vi "Begin.vi"(11 "Image Size":T1=enum."160x120") -> (0 "error out":errorcluster)   [LabVIEW 2012]
doc: "Called before other user functions, this VI is expected to open initial I/O refnums, load in file data, and do all program initialization. Notice that the <B>error out</B> terminal is simply used for data flow. Wiring it to other structures or subVIs ensures that this VI runs first."
uses:
  <vilib>/Rock Robotics/WPI/Camera/WPI_CameraImageSize.ctl
  <vilib>/Rock Robotics/SystemInterfaces/DIO/FPGA_DIOPWMChannel.ctl
  <vilib>/Rock Robotics/WPI/Joystick/WPI_JoystickDeviceEnum.ctl
  <vilib>/Rock Robotics/SystemInterfaces/DIO/FPGA_DIOChannel.ctl
  <vilib>/Rock Robotics/SystemInterfaces/AI/FPGA_AIGyroChannel.ctl
  <vilib>/Rock Robotics/WPI/Camera/WPI_CameraWhite Balance Values.ctl
  <vilib>/Rock Robotics/WPI/Camera/WPI_CameraExposure Values.ctl
  <vilib>/Rock Robotics/WPI/Camera/WPI_CameraFrameRate.ctl
  <vilib>/Rock Robotics/WPI/MotorControl/WPI_MotorControlOpen Victor.vi
  Robot Global Data.vi
  <vilib>/Rock Robotics/SystemInterfaces/Typedef/FPGA_TypedefDigitalModule.ctl
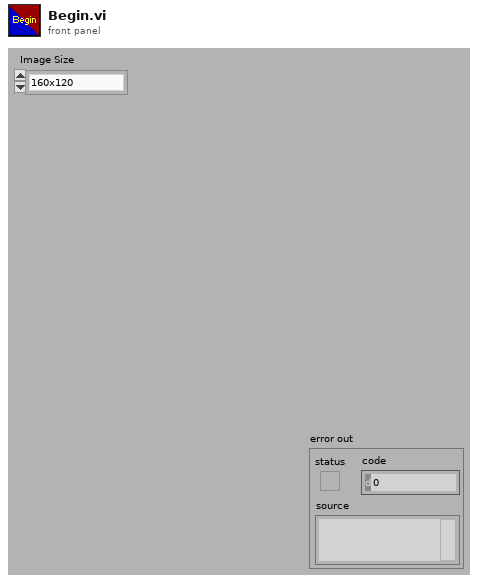
[diagram p1: front panel]
types:
  T1 = typedef "WPI_CameraImageSize.ctl" = enum16{"640x480", "320x240", "160x120"}
  T2 = typedef "FPGA_DIOPWMChannel.ctl" = enum8{"PWM 1", "PWM 2", "PWM 3", "PWM 4", "PWM 5", "PWM 6", "PWM 7", "PWM 8", "PWM 9", "PWM 10", "Invalid"}
  T3 = typedef "WPI_CameraFrameRate.ctl" = u32
  T4 = typedef "WPI_CameraExposure Values.ctl" = enum16{"Auto", "Flicker-free 50 Hz", "Flicker-free 60 Hz", "Hold current"}
  T5 = typedef "WPI_CameraWhite Balance Values.ctl" = enum16{"Auto", "Fixed indoor", "Fixed outdoor 1", "Fixed outdoor 2", "Fixed fluorescent 1", "Fixed fluorescent 2", "Hold current"}
  T6 = typedef "FPGA_AIGyroChannel.ctl" = enum8{"AI 1", "AI 2", "Invalid"}
  T7 = typedef "FPGA_DIOChannel.ctl" = enum8{"DIO 1", "DIO 2", "DIO 3", "DIO 4", "DIO 5", "DIO 6", "DIO 7", "DIO 8", "DIO 9", "DIO 10", "DIO 11", "DIO 12", "DIO 13", "DIO 14", "Invalid"}
  T8 = typedef "WPI_JoystickDeviceEnum.ctl" = enum16{"USB 1", "USB 2", "USB 3", "USB 4", "Kinect 1", "Kinect 2"}
  T9 = typedef "WPI_MotorControlDeviceRef.ctl" = cluster{"DeviceStatus":errorcluster, "Type":enum16{"PWM", "CAN"}, "PWM":cluster{"Digital Module":T10, "PWM Channel":T2, "DeadBand":T11}, "CAN":cluster{"Device Number":u8, "Control Mode":T12, "Semaphore":T13, "Max Vout":dbl}, "Invert":bool, "TransformRef":T14, "InvTransformRef":T14}
  T10 = typedef "FPGA_TypedefDigitalModule.ctl" = enum16{"Digital Module 1", "Digital Module 2"}
  T11 = typedef "WPI_PWMDeadband.ctl" = cluster{"Name":string, "maxPositivePwm":i32, "minPositivePwm":i32, "centerPwm":i32, "maxNegativePwm":i32, "minNegativePwm":i32, "angularRange":u16}
  T12 = typedef "WPI_CANJaguar_ControlMode.ctl" = enum8{"Percent VBus", "Current", "Speed", "Position", "Voltage"}
  T13 = typedef "Semaphore RefNum" = refnum<k1>
  T14 = typedef "WPI_PWMTransform_ConPane.ctl" = refnum<vi>
  T15 = typedef "WPI_CameraDevRef.ctl" = cluster{"Camera Address":string, "CameraStatus":errorcluster, "Acquire Image Notifier":refnum<notifier>}
  T16 = typedef "WPI_JoystickDevRef.ctl" = cluster{"Device":T8}
  T17 = typedef "WPI_ServoDeviceRef.ctl" = cluster{"DeviceStatus":errorcluster, "Digital Module":T10, "PWM Channel":T2, "DeadBand":T11}
  T18 = typedef "WPI_I2CDevRef.ctl" = cluster{"DevStatus":errorcluster, "Digital Module":T10, "Device Address":u8}
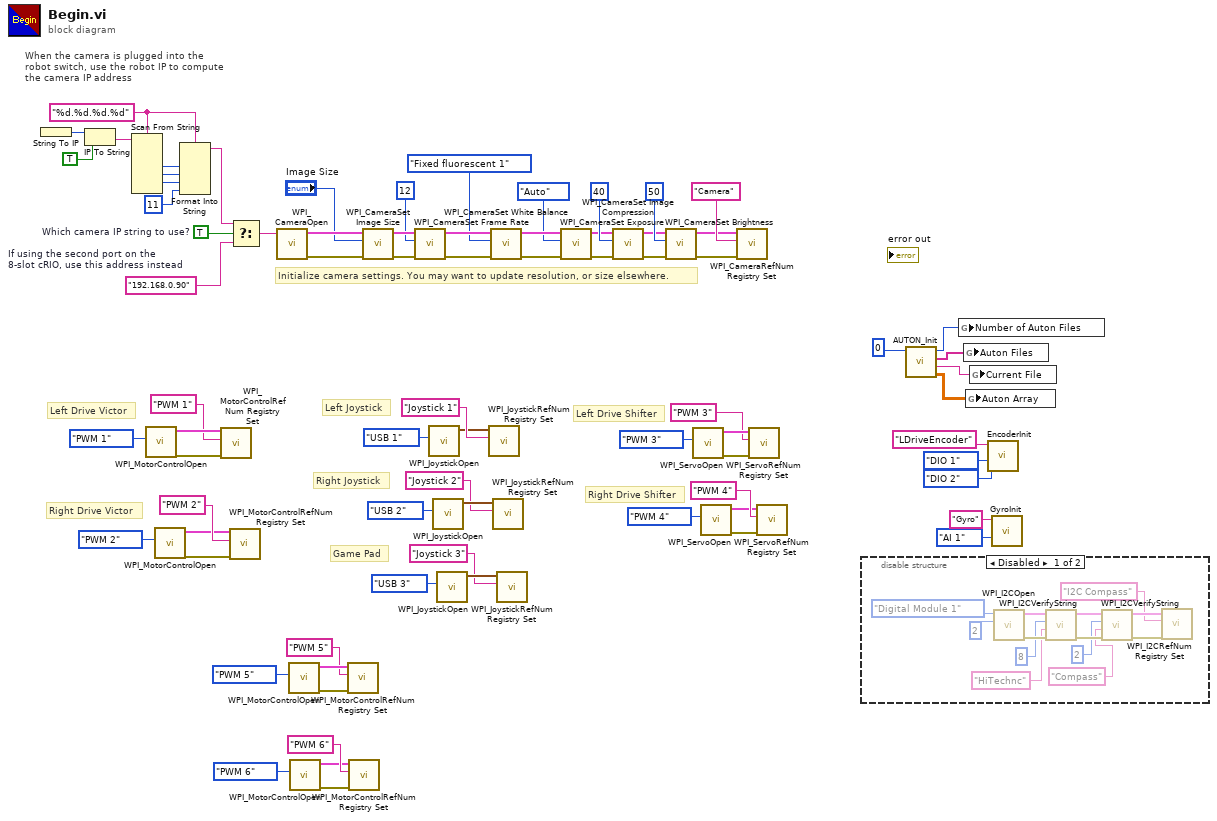
[diagram p0: block diagram]
diagram:
  w9 = TRUE  # Which camera IP string to use?
  w13 = "%d.%d.%d.%d" ("format string")
  w10 = "192.168.0.90"  # If using the second port on the 8-slot cRIO, use this address instead
  # "When the camera is plugged into the\nrobot switch, use the robot IP to compute\nthe camera IP address"
  # "Initialize camera settings. You may want to update resolution, or size elsewhere."
  # "Right Drive Shifter"
  # "Left Drive Shifter"
  # "Right Joystick"
  # "Left Joystick"
  # "Game Pad"
  # "Right Drive Victor"
  # "Left Drive Victor"
  n1 = String To IP() -> (0:w20:u32)  [unwired: 1 in]
  n2 = IP To String(1:TRUE ("dot notation? (F)"), 2:w20) -> (0:w18:string)
  n3 = Scan From String(format string=w13, input string=w18) -> (output 1=w17:i32, output 2=w16:i32, output 3=w15:i32)  [unwired: 7 in, 3 out]
  n4 = call-poly <vilib>:"WPI_MotorControlOpen.vi"("PWM Channel"=FPGA_DIOPWMChannel."PWM 1") -> ("error out"=w75:errorcluster, "MotorControlDeviceRef"=w76:T9)  [unwired: 9 in]
  n5 = call-poly <vilib>:"WPI_MotorControlOpen.vi"("PWM Channel"=FPGA_DIOPWMChannel."PWM 2") -> ("error out"=w70:errorcluster, "MotorControlDeviceRef"=w69:T9)  [unwired: 9 in]
  n6 = Format Into String(format string=w13, w17, w16, w15, 11 ("Compression")) -> (resulting string=w11:string)  [unwired: 2 in, 1 out]
  n7 = call <vilib>:"WPI_MotorControlRefNum Registry Set.vi"("error in (no error)"=w75, "refnum name"="PWM 1", "MotorControlDevRef"=w76) -> ()  [unwired: 7 in, 2 out]
  n8 = call <vilib>:"WPI_MotorControlRefNum Registry Set.vi"("error in (no error)"=w70, "refnum name"="PWM 2", "MotorControlDevRef"=w69) -> ()  [unwired: 7 in, 2 out]
  n9 = Select(t=w11, s=w9, f=w10) -> (s? t:f=w12:string)
  n10 = call <vilib>:"WPI_CameraOpen.vi"("Camera Address"=w12) -> ("error out"=w32:errorcluster, "CameraDevRef"=w33:T15)  [unwired: 1 in, 8 out]
  n11 = call-poly <vilib>:"WPI_MotorControlOpen.vi"("PWM Channel"=FPGA_DIOPWMChannel."PWM 5") -> ("error out"=w8:errorcluster, "MotorControlDeviceRef"=w7:T9)  [unwired: 9 in]
  n12 = call-poly <vilib>:"WPI_MotorControlOpen.vi"("PWM Channel"=FPGA_DIOPWMChannel."PWM 6") -> ("error out"=w1:errorcluster, "MotorControlDeviceRef"=w2:T9)  [unwired: 9 in]
  n13 = call <vilib>:"WPI_MotorControlRefNum Registry Set.vi"("error in (no error)"=w8, "refnum name"="PWM 5", "MotorControlDevRef"=w7) -> ()  [unwired: 7 in, 2 out]
  n14 = call <vilib>:"WPI_MotorControlRefNum Registry Set.vi"("error in (no error)"=w1, "refnum name"="PWM 6", "MotorControlDevRef"=w2) -> ()  [unwired: 7 in, 2 out]
  n15 = call <vilib>:"WPI_CameraSet Image Size.vi"("error in (no error)"=w32, "Image Size"="Image Size", "CameraDevRef"=w33) -> ("error out"=w31:errorcluster, "CameraDevRef Out"=w34:T15)  [unwired: 7 out]
  n16 = call <vilib>:"WPI_CameraSet Frame Rate.vi"("error in (no error)"=w31, "Frame Rate (fps)"=T3 12, "CameraDevRef"=w34) -> ("error out"=w30:errorcluster, "CameraDevRef Out"=w36:T15)  [unwired: 7 out]
  n17 = call <vilib>:"WPI_JoystickOpen.vi"("JoystickDevice"=WPI_JoystickDeviceEnum."USB 1") -> ("JoystickDevRef"=w60:T16)  [unwired: 10 in]
  n18 = call <vilib>:"WPI_JoystickOpen.vi"("JoystickDevice"=WPI_JoystickDeviceEnum."USB 2") -> ("JoystickDevRef"=w65:T16)  [unwired: 10 in]
  n19 = call <vilib>:"WPI_JoystickOpen.vi"("JoystickDevice"=WPI_JoystickDeviceEnum."USB 3") -> ("JoystickDevRef"=w68:T16)  [unwired: 10 in]
  n20 = call <vilib>:"WPI_JoystickRefNum Registry Set.vi"("refnum name"="Joystick 1", "JoystickDevRef"=w60) -> ()  [unwired: 8 in, 2 out]
  n21 = call <vilib>:"WPI_CameraSet White Balance.vi"("error in (no error)"=w30, "White Balance"=WPI_CameraWhite_Balance_Values."Fixed fluorescent 1", "CameraDevRef"=w36) -> ("error out"=w29:errorcluster, "CameraDevRef Out"=w35:T15)  [unwired: 7 out]
  n22 = call <vilib>:"WPI_JoystickRefNum Registry Set.vi"("refnum name"="Joystick 2", "JoystickDevRef"=w65) -> ()  [unwired: 8 in, 2 out]
  n23 = call <vilib>:"WPI_JoystickRefNum Registry Set.vi"("refnum name"="Joystick 3", "JoystickDevRef"=w68) -> ()  [unwired: 8 in, 2 out]
  n24 = call <vilib>:"WPI_CameraSet Exposure.vi"("error in (no error)"=w29, "Exposure"=WPI_CameraExposure_Values."Auto", "CameraDevRef"=w35) -> ("error out"=w28:errorcluster, "CameraDevRef Out"=w38:T15)  [unwired: 7 out]
  n25 = call <vilib>:"WPI_CameraSet Image Compression.vi"("error in (no error)"=w28, "Compression"=40, "CameraDevRef"=w38) -> ("error out"=w27:errorcluster, "CameraDevRef Out"=w37:T15)  [unwired: 7 out]
  n26 = call <vilib>:"WPI_CameraSet Brightness.vi"("error in (no error)"=w27, "Brightness"=50, "CameraDevRef"=w37) -> ("error out"=w25:errorcluster, "CameraDevRef Out"=w26:T15)  [unwired: 7 out]
  n27 = call <vilib>:"WPI_ServoOpen.vi"("PWM Channel"=FPGA_DIOPWMChannel."PWM 3") -> ("error out"=w59:errorcluster, "ServoDeviceRef"=w58:T17)  [unwired: 9 in]
  n28 = call <vilib>:"WPI_ServoOpen.vi"("PWM Channel"=FPGA_DIOPWMChannel."PWM 4") -> ("error out"=w52:errorcluster, "ServoDeviceRef"=w53:T17)  [unwired: 9 in]
  n29 = call <vilib>:"WPI_CameraRefNum Registry Set.vi"("error in (no error)"=w25, "refnum name"="Camera", "CameraDevRef"=w26) -> ()  [unwired: 9 out]
  n30 = call <vilib>:"WPI_ServoRefNum Registry Set.vi"("error in (no error)"=w59, "refnum name"="PWM 3", "ServoDeviceRef"=w58) -> ()  [unwired: 7 in, 2 out]
  n31 = call <vilib>:"WPI_ServoRefNum Registry Set.vi"("error in (no error)"=w52, "refnum name"="PWM 4", "ServoDeviceRef"=w53) -> ()  [unwired: 7 in, 2 out]
  n32 = disable-structure shown="Disabled" {
    frame Disabled {
      n33 = call <vilib>:"WPI_I2COpen.vi"("Device Address"=u8 2, "Digital Module (Module 1)"=FPGA_TypedefDigitalModule."Digital Module 1") -> ("error out"=w89:errorcluster, "I2CDevRef"=w88:T18)  [unwired: 8 in]
      n34 = call <vilib>:"WPI_I2CVerifyString.vi"("error in (no error)"=w89, "Expected"="HiTechnc", "Register Address"=u8 8, "I2CDevRef"=w88) -> ("error out"=w87:errorcluster, "I2CDevRef"=w86:T18)  [unwired: 6 in]
      n35 = call <vilib>:"WPI_I2CVerifyString.vi"("error in (no error)"=w87, "Expected"="Compass", "Register Address"=u8 2, "I2CDevRef"=w86) -> ("error out"=w85:errorcluster, "I2CDevRef"=w84:T18)  [unwired: 6 in]
      n36 = call <vilib>:"WPI_I2CRefNum Registry Set.vi"("error in (no error)"=w85, "refnum name"="I2C Compass", "I2CDevRef"=w84) -> ()  [unwired: 7 in, 2 out]
    }
    frame Enabled {
    }
  }
  n37 = call "AUTON_Init.vi"("Default File"=0) -> ("Auton Array"=w49:dbl[][], "Current File"=w48:string, "Auton Files"=w50:string[], "Number of Auton Files"=w51:i64)  [unwired: 7 in]
  n38 = global write "Robot Global Data.vi" "Number of Auton Files"(w51) -> ()
  n39 = global write "Robot Global Data.vi" "Auton Files"(w50) -> ()
  n40 = global write "Robot Global Data.vi" "Auton Array"(w49) -> ()
  n41 = global write "Robot Global Data.vi" "Current File"(w48) -> ()
  n42 = call "EncoderInit.vi"("refnum name"="LDriveEncoder", "DIO Channel"=FPGA_DIOChannel."DIO 1", "DIO Channel 2"=FPGA_DIOChannel."DIO 2") -> ()  [unwired: 8 in]
  n43 = call "GyroInit.vi"("refnum name"="Gyro", "Analog Channel"=FPGA_AIGyroChannel."AI 1") -> ()  [unwired: 8 in]
